vi "add_txt_all.vi"   [LabVIEW 2016]
types:
  T1 = enum16{"open", "replace", "create", "open or create", "replace or create", "replace or create with confirmation"}
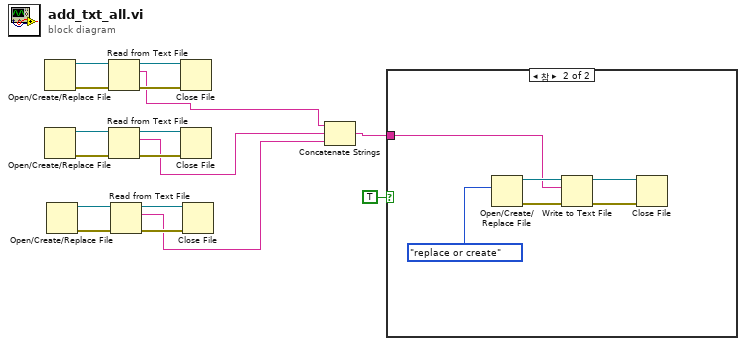
[diagram p0: block diagram]
diagram:
  n1 = Open/Create/Replace File() -> (refnum out=w14:refnum<file>, error out=w17:errorcluster)  [unwired: 6 in, 1 out]
  n2 = Open/Create/Replace File() -> (refnum out=w13:refnum<file>, error out=w10:errorcluster)  [unwired: 6 in, 1 out]
  n3 = Open/Create/Replace File() -> (refnum out=w6:refnum<file>, error out=w9:errorcluster)  [unwired: 6 in, 1 out]
  n4 = Read from Text File(file (use dialog)=w14, error in=w17) -> (refnum out=w15:refnum<file>, text=w5:string, error out=w16:errorcluster)  [unwired: 2 in, 1 out]
  n5 = Read from Text File(file (use dialog)=w13, error in=w10) -> (refnum out=w12:refnum<file>, text=w4:string, error out=w11:errorcluster)  [unwired: 2 in, 1 out]
  n6 = Read from Text File(file (use dialog)=w6, error in=w9) -> (refnum out=w7:refnum<file>, text=w3:string, error out=w8:errorcluster)  [unwired: 2 in, 1 out]
  n7 = Close File(refnum=w15, error in=w16) -> ()  [unwired: 2 out]
  n8 = Close File(refnum=w12, error in=w11) -> ()  [unwired: 2 out]
  n9 = Close File(refnum=w7, error in=w8) -> ()  [unwired: 2 out]
  n10 = Concatenate Strings(w5, w4, w3) -> (w2:string)
  n11 = case shown="참" TRUE {
    tunnel: w2 -> [_ w18]
    frame False {
    }
    frame True {
      n12 = Open/Create/Replace File(operation (0:open)=T1."replace or create" ("동작(0:open)")) -> (refnum out=w20:refnum<file>, error out=w21:errorcluster)  [unwired: 5 in, 1 out]
      n13 = Write to Text File(file (use dialog)=w20, text=w18, error in=w21) -> (refnum out=w23:refnum<file>, error out=w22:errorcluster)  [unwired: 1 in, 1 out]
      n14 = Close File(refnum=w23, error in=w22) -> ()  [unwired: 2 out]
    }
  }
